vi "周期设置_总磷总氮.vi"() -> ()   [LabVIEW 2016, in "斯坦道氨氮.lvlib"]
uses:
  <vilib>/Utility/miscctls.llb/LVPointTypeDef.ctl
panel:
  in  "运行周期":T1={"运行模式"=enum."维护模式", "质控频次"=enum."关闭", "空白核查时间"=2, "跨度核查时间"=6, "24H周期设置"=[]} {"跨度核查时间" items=["00H", "01H", "02H", "03H", "04H", "05H", "06H", "07H", "08H", "09H", "10H", "11H", "12H", "13H", "14H", "15H", "16H", "17H", "18H", "19H", "20H", "21H", "22H", "23H", "关闭"]; "空白核查时间" items=["00H", "01H", "02H", "03H", "04H", "05H", "06H", "07H", "08H", "09H", "10H", "11H", "12H", "13H", "14H", "15H", "16H", "17H", "18H", "19H", "20H", "21H", "22H", "23H", "关闭"]}
  # "运行模式："
  # "质控频次："
  # "零点核查时间："
  # "跨度核查时间："
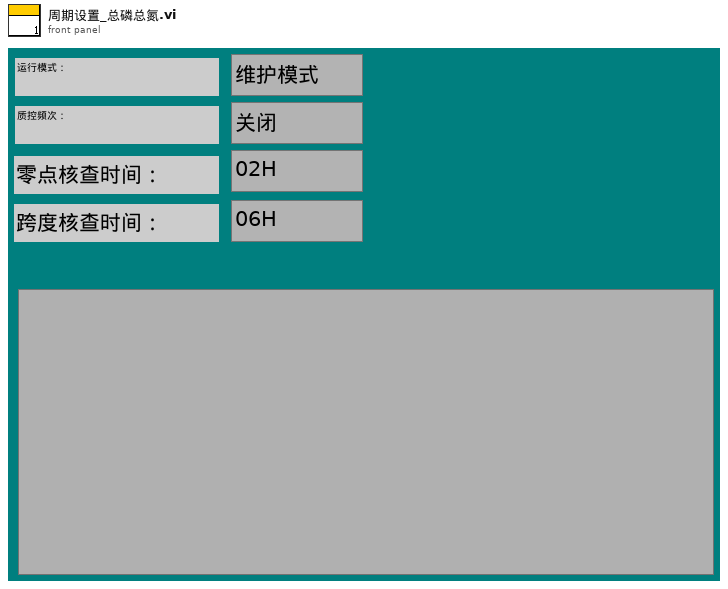
[diagram p1: front panel]
types:
  T1 = cluster{"运行模式":enum16{"维护模式", "常规模式", "应急模式", "质控模式"}, "质控频次":enum16{"关闭", "每天", "星期一", "星期二", "星期三", "星期四", "星期五", "星期六", "星期日"}, "空白核查时间":u16, "跨度核查时间":u16, "24H周期设置":bool[]}
  T2 = typedef "LVPointTypeDef.ctl" = cluster{"Horizontal":i16, "Vertical":i16}
  T3 = enum16{"启动测量", "标样核查", "零点核查", "跨度核查", "空白测试", "平行样测试", "加标回收", "空白校准", "标样校准", "初始化（清洗）", "停止测试", "仪器重启", "校时", "模式设置", "测量间隔设置"}
  T4 = cluster{"系统时间":timestamp, "工作状态":u16, "测量模式":enum16{"待机", "连续模式", "周期模式", "定点模式", "受控模式", "手动模式"}, "告警代码":u16, "故障代码":u16, "日志代码":u16, "软件版本":u16, "F0":sgl, "F1":sgl, "F2":sgl, "F3":sgl, "T":sgl, "H":sgl, "id":u16, "flowid":u16, "量程":u16, "总磷控温温度1":sgl, "营养盐控温温度2":sgl, "ADC":sgl}
  T5 = enum16{"关闭", "每天", "星期一", "星期二", "星期三", "星期四", "星期五", "星期六", "星期日"}
  T6 = typedef "LVDateTimeRec.ctl" = cluster{"秒数的小数部分":dbl, "秒":i32, "分":i32, "时":i32, "日":i32, "月":i32, "年":i32, "天数（周）":i32, "天数（年）":i32, "DST":i32}
  T7 = enum32{"Bad", "Idle", "Run top level", "Running"}
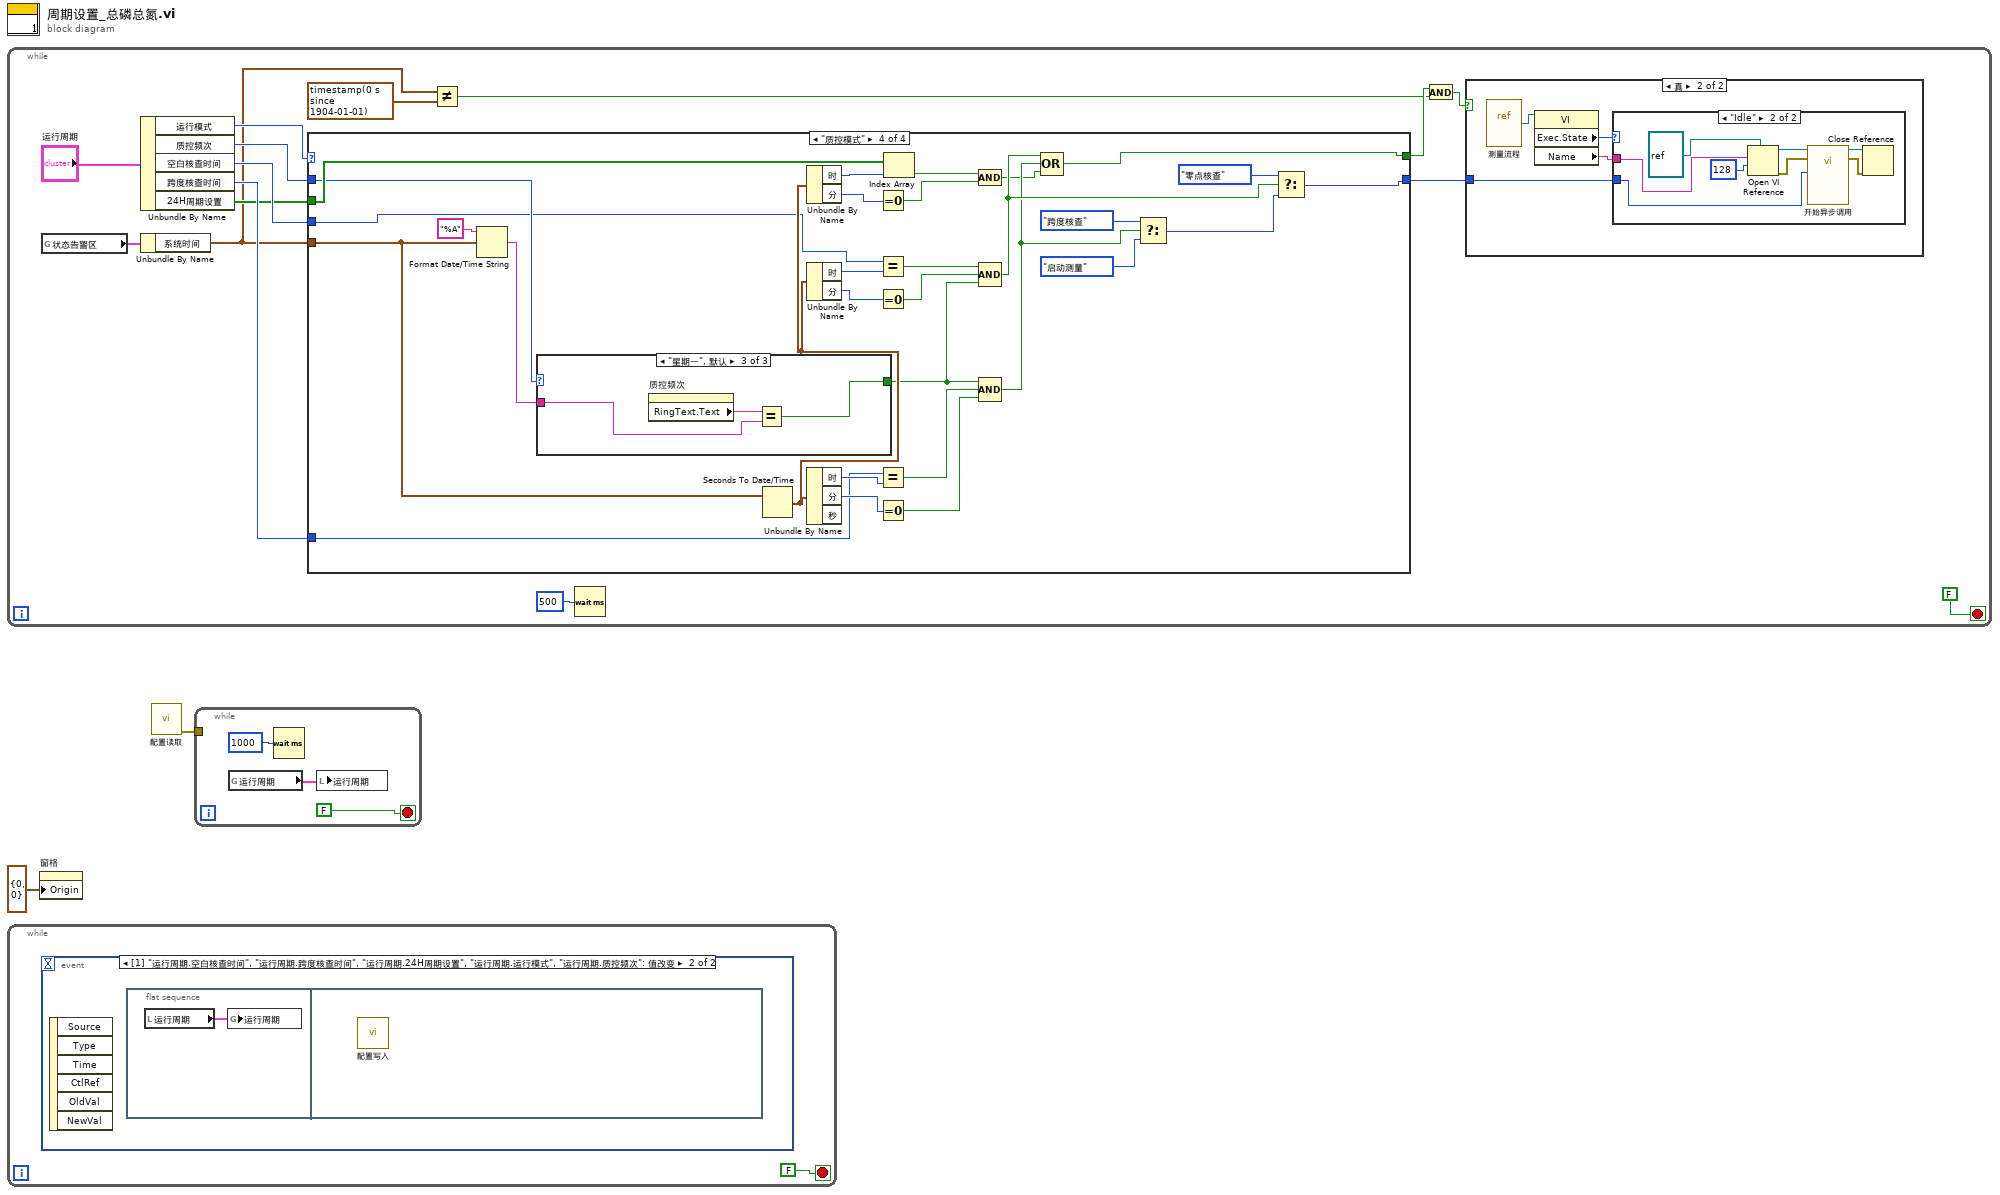
[diagram p0: block diagram]
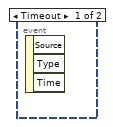
[diagram p2: hidden frame]
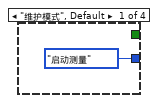
[diagram p5: hidden frame]
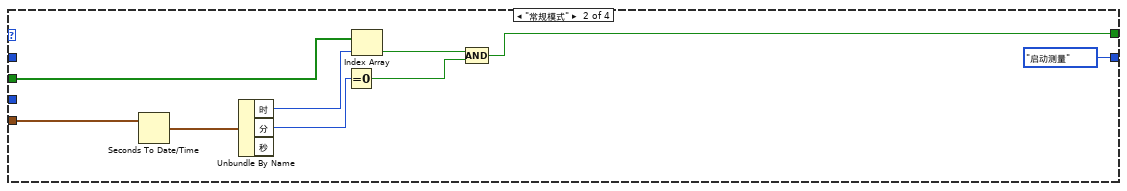
[diagram p6: hidden frame]
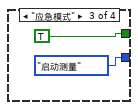
[diagram p7: hidden frame]
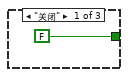
[diagram p8: hidden frame]
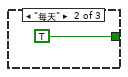
[diagram p9: hidden frame]
diagram:
  n1 = while {
    stop <- FALSE stop-if-true
    n2 = global read "VAR总磷总氮全局变量.vi" "状态告警区"() -> (w7:T4)
    n3 = Unbundle By Name("运行周期") -> ("运行模式"=w14:enum16{"维护模式", "常规模式", "应急模式", "质控模式"}, "质控频次"=w13:T5, "空白核查时间"=w12:u16, "跨度核查时间"=w11:u16, "24H周期设置"=w10:bool[])
    n4 = Unbundle By Name(w7) -> ("系统时间"=w6:timestamp)
    n5 = case shown="\"质控模式\"" w14 {
      tunnel: w6 -> [_ w39 _ w71]
      tunnel: w10 -> [_ w36 _ w68]
      tunnel: [_ w32 TRUE w54] -> w9
      tunnel: [T3."启动测量" ("控制命令") T3."启动测量" ("控制命令") T3."启动测量" ("控制命令") w50] -> w8
      tunnel: w13 -> [_ _ _ w47]
      tunnel: w12 -> [_ _ _ w46]
      tunnel: w11 -> [_ _ _ w45]
      frame "维护模式", Default {
      }
      frame "常规模式" {
        n6 = Seconds To Date/Time(time stamp (now)=w39) -> (date time rec=w38:T6)  [unwired: 1 in]
        n7 = Unbundle By Name(w38) -> ("时"=w37:i32, "分"=w35:i32)  [unwired: 1 out]
        n8 = Equal To 0?(x=w35) -> (x = 0?=w33:bool)
        n9 = Index Array(array=w36, index=w37) -> (element=w34:bool)
        n10 = Compound Arithmetic op=AND ("复合运算")(w34, w33) -> (w32:bool)
      }
      frame "应急模式" {
      }
      frame "质控模式" {
        n11 = Format Date/Time String(time format string (%c)="%A" ("时间格式字符串(%c)"), seconds (now)=w71) -> (date/time string=w69:string)  [unwired: 1 in]
        n12 = case shown="\"星期一\", 默认" w47 {
          tunnel: w69 -> [_ _ w75]
          tunnel: [FALSE TRUE w74] -> w48
          frame "关闭" {
          }
          frame "每天" {
          }
          frame "星期一", Default {
            n13 = property on="质控频次" class="Enum (严格)"() -> ("RingText.Text"=w76:string)  [unwired: 2 in, 2 out]
            n14 = Equal?(x=w76, y=w75) -> (x = y?=w74:bool)
          }
        }
        n15 = Seconds To Date/Time(time stamp (now)=w71) -> (date time rec=w57:T6)  [unwired: 1 in]
        n16 = Unbundle By Name(w57) -> ("时"=w67:i32, "分"=w65:i32)
        n17 = Unbundle By Name(w57) -> ("时"=w63:i32, "分"=w62:i32)
        n18 = Unbundle By Name(w57) -> ("时"=w58:i32, "分"=w59:i32)  [unwired: 1 out]
        n19 = Equal To 0?(x=w65) -> (x = 0?=w64:bool)
        n20 = Equal?(x=w46, y=w63) -> (x = y?=w61:bool)
        n21 = Equal To 0?(x=w62) -> (x = 0?=w60:bool)
        n22 = Equal?(x=w45, y=w58) -> (x = y?=w56:bool)
        n23 = Equal To 0?(x=w59) -> (x = 0?=w55:bool)
        n24 = Index Array(array=w68, index=w67) -> (element=w66:bool)
        n25 = Compound Arithmetic op=AND ("复合运算")(w66, w64) -> (w49:bool)
        n26 = Compound Arithmetic op=AND ("复合运算")(w61, w60, w48) -> (w53:bool)
        n27 = Compound Arithmetic op=AND ("复合运算")(w48, w56, w55) -> (w52:bool)
        n28 = Compound Arithmetic op=OR ("复合运算")(w53, w52, w49) -> (w54:bool)
        n29 = Select(t=T3."跨度核查" ("控制命令"), s=w52, f=T3."启动测量" ("控制命令")) -> (s? t:f=w51:T3)
        n30 = Select(t=T3."零点核查" ("控制命令"), s=w53, f=w51) -> (s? t:f=w50:T3)
      }
    }
    n31 = Not Equal?(x=w6, y=timestamp(0 s since 1904-01-01)) -> (x != y?=w3:bool)
    n32 = Wait (ms)(milliseconds to wait=u32 500 ("等待时间（毫秒）")) -> ()  [unwired: 1 out]
    n33 = And(x=w9, y=w3) -> (x .and. y?=w4:bool)
    n34 = case shown="真" w4 {
      tunnel: w8 -> [_ w19]
      frame False {
      }
      frame True {
        n35 = vi-ref "测量流程.vi"() -> (w20:refnum<vi>)
        n36 = property class="VI"(reference=w20) -> ("Exec.State"=w18:T7, "Name"=w21:string)  [unwired: 1 in, 2 out]
        n37 = case shown="\"Idle\"" w18 {
          tunnel: w21 -> [_ w25]
          tunnel: w19 -> [_ w22]
          frame "Bad", Default {
          }
          frame "Idle" {
            n38 = Open VI Reference(type specifier VI Refnum (for type only)=refnum<vi> refnum, vi path=w25, options=128 ("选项")) -> (vi reference=w26:refnum<vi>, error out=w27:errorcluster)  [unwired: 3 in]
            n39 = call-by-ref "开始异步调用"(reference=w26, error in=w27, "控制命令"=w22) -> (reference out=w28:refnum<vi>, error out=w29:errorcluster)  [unwired: 11 in]
            n40 = Close Reference(reference=w28, error in (no error)=w29) -> ()  [unwired: 1 out]
          }
        }
      }
    }
  }
  n41 = while {
    stop <- FALSE stop-if-true
    n42 = event shown="[1] \"运行周期.空白核查时间\", \"运行周期.跨度核查时间\", \"运行周期.24H周期设置\", \"运行周期.运行模式\", \"运行周期.质控频次\": 值改变" {
      selector: _ -> [_ _]
      dyn-events: _ -> [_ _]
      timeout: _ -> [_ _]
      event Timeout {
        n43 = event-data() -> ()  [unwired: 1 in, 3 out]
      }
      event "运行周期.空白核查时间", "运行周期.跨度核查时间", "运行周期.24H周期设置", "运行周期.运行模式", "运行周期.质控频次": Value Change {
        n44 = event-data() -> ()  [unwired: 1 in, 6 out]
        n45 = flat-sequence {
          frame #0 {
            n46 = local read "运行周期"() -> (w78:T1)
            n47 = global write "总磷总氮断电保存全局变量.vi" "运行周期"(w78) -> ()
          }
          frame #1 {
            n48 = call "配置写入.vi"() -> ()  [unwired: 11 in, 1 out]
          }
        }
      }
    }
  }
  n49 = property on="窗格" class="Pane"("Origin"=T2 {"Horizontal"=0, "Vertical"=0} ("原点")) -> ()  [unwired: 2 in, 2 out]
  n50 = call "配置读取.vi"() -> ("error out"=w1:errorcluster)  [unwired: 11 in]
  n51 = while {
    tunnel: w1 -> [_]
    stop <- FALSE stop-if-true
    n52 = global read "总磷总氮断电保存全局变量.vi" "运行周期"() -> (w79:T1)
    n53 = Wait (ms)(milliseconds to wait=u32 1000 ("等待时间（毫秒）")) -> ()  [unwired: 1 out]
    n54 = local write "运行周期"(w79) -> ()
  }
